vi "Fast_sampling_Ocean.vi"() -> ()   [LabVIEW 2022 SP3]
panel:
  in  "Numeric":i32
  in  "Integration Time (us)":dbl=10000.0
  out "Number of Spectrometers":i32
  out "?":T1(graph)
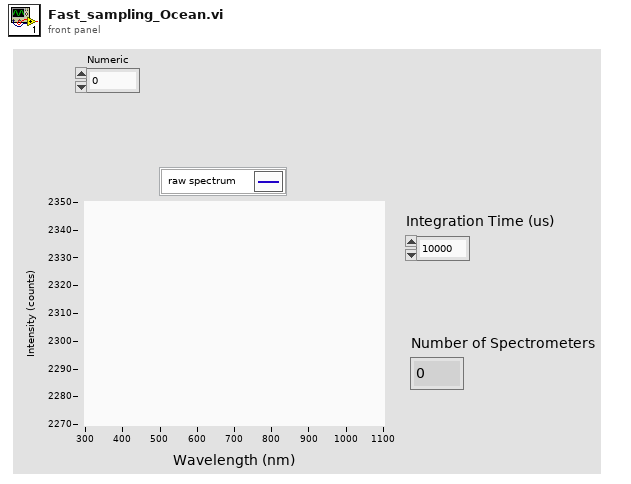
[diagram p1: front panel]
types:
  T1 = cluster{"WL Values":dbl[], "Spectrum Values":dbl[]}
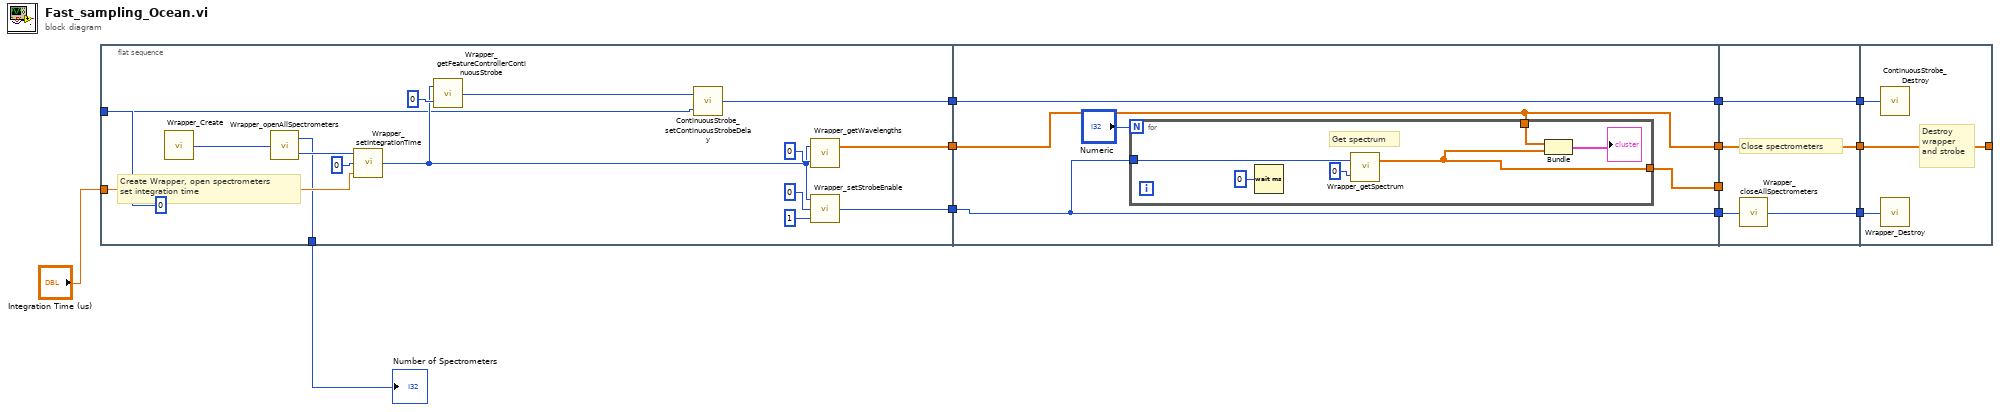
[diagram p0: block diagram]
diagram:
  n1 = flat-sequence {
    tunnel: [w19] -> w13
    tunnel: [w18] -> w12
    tunnel: [w17] -> w11
    tunnel: "Integration Time (us)" -> [w16]
    tunnel: [w15] -> w3
    tunnel: 0 ("Continuous \nStrobe Delay") -> [w14]
    tunnel: [w33] -> w10
    tunnel: w13 -> [w33]
    tunnel: w12 -> [w29]
    tunnel: [w29] -> w9
    tunnel: w11 -> [w32]
    tunnel: [w32] -> w8
    tunnel: [w31] -> w7
    tunnel: [w43] -> w6
    tunnel: w10 -> [w43]
    tunnel: w9 -> [w42]
    tunnel: [w41] -> w5
    tunnel: [w40] -> w4
    tunnel: w8 -> [w40]
    tunnel: w7 -> [_]
    tunnel: w6 -> [w46]
    tunnel: w5 -> [w45]
    tunnel: [w44] -> _
    tunnel: w4 -> [w44]
    frame #0 {
      # "Create Wrapper, open spectrometers\nset integration time"
      n2 = call "Wrapper_Create.vi"() -> ("Wrapper"=w28:u32)
      n3 = call "Wrapper_openAllSpectrometers.vi"("Wrapper In"=w28) -> ("Number of Spectrometers"=w15:i32, "Wrapper Out"=w22:u32)
      n4 = call "Wrapper_setIntegrationTime.vi"("Integration Time"=w16, "Spectrometer Index"=0 ("Index"), "Wrapper In"=w22) -> ("Wrapper Out"=w20:u32)
      n5 = call "Wrapper_getFeatureControllerContinuousStrobe.vi"("Index"=0, "Wrapper"=w20) -> ("ContinuousStrobe"=w25:u32)
      n6 = call "ContinuousStrobe_setContinuousStrobeDelay.vi"("delay"=w14, "ContinuousStrobe In"=w25) -> ("ContinuousStrobe Out"=w19:u32)
      n7 = call "Wrapper_getWavelengths.vi"("Index"=0, "Wrapper"=w20) -> ("WL Values"=w17:dbl[])  [unwired: 1 out]
      n8 = call "Wrapper_setStrobeEnable.vi"("On/Off"=1, "Index"=0, "Wrapper In"=w20) -> ("Wrapper Out"=w18:u32)
    }
    frame #1 {
      n9 = for {
        N: "Numeric" -> [_]
        tunnel: w29 -> [w39]
        tunnel: [w37] -> w31
        tunnel: w32 -> [w36]
        # "Get spectrum"
        n10 = Wait (ms)(milliseconds to wait=u32 0) -> ()  [unwired: 1 out]
        n11 = call "Wrapper_getSpectrum.vi"("Index"=0, "Wrapper"=w39) -> ("Spectrum Values"=w37:dbl[])  [unwired: 1 out]
        n12 = Bundle("WL Values"=w36, "Spectrum Values"=w37) -> (→"?":T1)  [unwired: 1 in]
      }
    }
    frame #2 {
      # "Close spectrometers"
      n13 = call "Wrapper_closeAllSpectrometers.vi"("Wrapper In"=w42) -> ("Wrapper Out"=w41:u32)
    }
    frame #3 {
      # "Destroy \nwrapper \nand strobe"
      n14 = call "ContinuousStrobe_Destroy.vi"("ContinuousStrobe"=w46) -> ()
      n15 = call "Wrapper_Destroy.vi"("Wrapper"=w45) -> ()
    }
  }
  "Number of Spectrometers" <- w3
